vi "SV FFT Spectrum (Mag-Phase).vi"(0 "scaled signal [EU]":dbl[](array[numeric]) format="%.2f", 1 "frequency weighting":T5(ring), 5 "sampling frequency [Hz]":dbl=10000.0 format="%.2f", 9 "window":T6 items=["Rectangle"=0, "Hanning"=1, "Hamming"=2, "Blackman-Harris"=3, "Exact Blackman"=4, "Blackman"=5, "Flat Top"=6, "4 Term B-Harris "=7, "7 Term B-Harris"=8, "Low Sidelobe"=9, "Blackman Nuttall"=11, "Triangle"=30, "Bartlett-Hanning"=31, "Bohman"=32, "Parzen"=33, "Welch"=34, "Kaiser"=60, "Dolph-Chebyshev"=61, "Gaussian"=62], 11 "channel info":T1={"sensor sensitivity [mV/EU]"=1000.0, "engineering units"=1, "dB reference [EU]"=1.0, "custom label"="EU", "weighting filter"=0, "pregain [dB]"=0.0} {"pregain [dB]" format="%.2f"; "weighting filter" items=["Linear", "A-weighting", "B-weighting", "C-weighting", "ITU-R 468-4", "Dolby", "CCITT", "C-message"]; "dB reference [EU]" format="%^.1e"; "engineering units" items=["custom..."=0, "V"=1, "A"=21, "Pa"=2, "N"=20, "g"=3, "m/s^2"=4, "m/s"=5, "m"=6, "mm/s"=12, "mm"=13, "microns/s"=14, "microns"=15, "in/s^2"=7, "in/s"=8, "in"=9, "mils/s"=10, "mils"=11, "rad/s^2"=16, "rad/s"=17, "rad"=18, "strain"=19]; "sensor sensitivity [mV/EU]" format="%.2f"}, 12 "view":T4) -> (3 "df [Hz]":dbl format="%.2f", 4 "magnitude [EUrms]":dbl[](array[numeric]) format="%.2f", 6 "unit label (magnitude)":string, 8 "phase":dbl[](array[numeric]) format="%.2f", 10 "unit label (phase)":string, 14 "window constants":cluster{"eq noise BW":dbl, "coherent gain":dbl} {"coherent gain" format="%.2f"; "eq noise BW" format="%.2f"}, 15 "weighting conflict":bool)   [LabVIEW 2017]
doc: "SV (Sound & Vibration) FFT Spectrum (Mag-Phase) computes the FFT spectrum of the input signal. FFT results are returned as magnitude and phase.\nThe view cluster allows you to display magnitude results in decibels, and the phase results unwrapped or not, in radians or degrees.\nThe selected frequency weighting (A, B, or C) is applied to the results in the frequency domain. There is no time-domain filtering operation."
uses:
  <vilib>/Analysis/4window.llb/windowTd.ctl
  <vilib>/addons/Sound and Vibration/compatibility/Controls/svl_Channel Info.ctl
  <vilib>/addons/Sound and Vibration/compatibility/Controls/svl_Engineering Units Text Ring.ctl
  <vilib>/addons/Sound and Vibration/compatibility/Controls/svl_Weighting Filter Text Ring.ctl
  <vilib>/Analysis/2dsp.llb/Real FFT.vi
  <vilib>/Analysis/0measdsp.llb/Scaled Time Domain Window (DBL).vi
  <vilib>/Analysis/NI_AALPro.lvlib
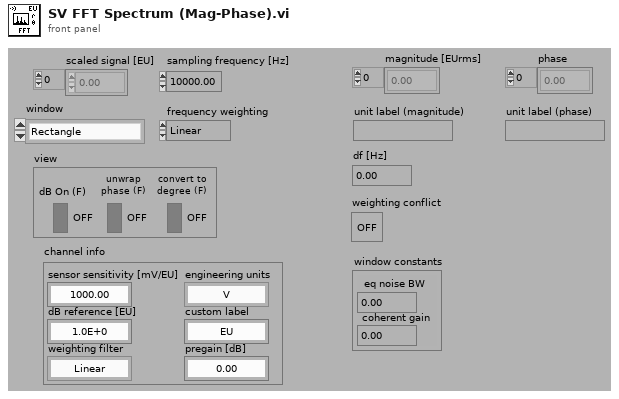
[diagram p1: front panel]
types:
  T1 = typedef "svl_Channel Info.ctl" = cluster{"sensor sensitivity [mV/EU]":dbl, "engineering units":T2, "dB reference [EU]":dbl, "custom label":string, "weighting filter":T3, "pregain [dB]":dbl}
  T2 = typedef "svl_Engineering Units Text Ring.ctl" = u16
  T3 = typedef "svl_Weighting Filter Text Ring.ctl" = u16
  T4 = cluster{"dB On (F)":bool, "unwrap phase (F)":bool, "convert to degree (F)":bool}
  T5 = enum16{"Linear", "A-weighting", "B-weighting", "C-weighting"}
  T6 = typedef "NI_AALPro.lvlib/windowTd.ctl" = u32
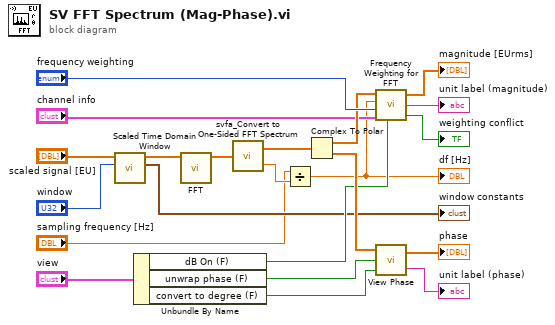
[diagram p0: block diagram]
diagram:
  n1 = call-poly <vilib>:"Scaled Time Domain Window.vi"("window"="window", "X"="scaled signal [EU]") -> ("window properties"=→"window constants":cluster{"eq noise BW":dbl, "coherent gain":dbl}, "Windowed X"=w4:dbl[])  [unwired: 7 in, 1 out]
  n2 = Unbundle By Name("view") -> ("dB On (F)"=w11:bool, "unwrap phase (F)"=w12:bool, "convert to degree (F)"=w13:bool)
  n3 = call-poly <vilib>:"FFT.vi"("X"=w4) -> ("FFT {X}"=w5:cdb[])  [unwired: 9 in, 1 out]
  n4 = call <vilib>:"svfa_Convert to One-Sided FFT Spectrum.vi"("two-sided FFT spectrum"=w5) -> ("one-sided FFT spectrum"=w2:cdb[], "block size"=w6:dbl)
  n5 = Divide(x="sampling frequency [Hz]", y=w6) -> (x/y=w1:dbl)
  "df [Hz]" <- w1
  n6 = Complex To Polar(r * e^(i*theta)=w2) -> (r=w16:dbl[], theta=w15:dbl[])
  n7 = call <vilib>:"Frequency Weighting for FFT.vi"("FFT [EUrms]"=w16, "df [Hz]"=w1, "frequency weighting"="frequency weighting", "channel info"="channel info", "dB On (F)"=w11) -> ("frequency weighted FFT [EUrms]"=→"magnitude [EUrms]":dbl[], "unit label"=→"unit label (magnitude)":string, "weighting conflict"=→"weighting conflict":bool)
  n8 = call <vilib>:"View Phase.vi"("convert to degree (F)"=w13, "unwrap phase (F)"=w12, "phase (radian)"=w15) -> ("unit label (phase)"=→"unit label (phase)":string, "scaled phase"=→"phase":dbl[])
